vi "Change Position.vi"(1 "Y Change":dbl, 2 "X Change":dbl, 3 "Car.lvclass":refnum<class "Car.lvclass">) -> (0 "Car.lvclass 2":refnum<class "Car.lvclass">)   [LabVIEW 2015, in "Car.lvclass"]
uses:
  Car.lvclass
  Car.lvclass/Car.ctl
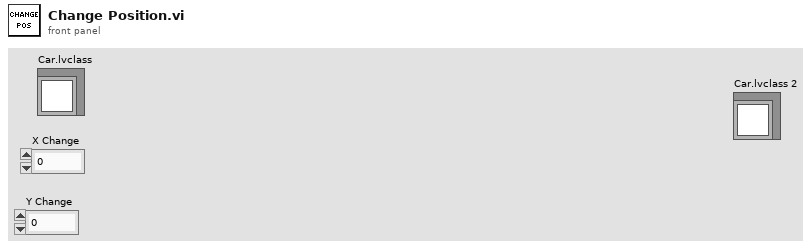
[diagram p1: front panel]
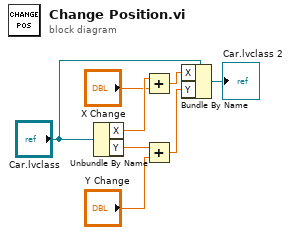
[diagram p0: block diagram]
diagram:
  n1 = Unbundle By Name("Car.lvclass") -> ("X"=w7:dbl, "Y"=w5:dbl)
  n2 = Add(x=w7, y="X Change") -> (x+y=w3:dbl)
  n3 = Add(x=w5, y="Y Change") -> (x+y=w2:dbl)
  n4 = Bundle By Name(cluster="Car.lvclass", "X"=w3, "Y"=w2) -> (→"Car.lvclass 2":refnum<class "Car.lvclass">)
